vi "Robot_Arduino_1.vi"() -> ()   [LabVIEW 2013]
uses:
  <vilib>/Utility/inputDevices.llb/closeJoystick.vi
  <vilib>/LabVIEW Hacker/LINX/LVH-LINX.lvlib
panel:
  out "Ultrasonic":dbl
  out "Switch":bool
  in  "Serial Port":refnum<visa-resource-name>
  in  "stop":bool
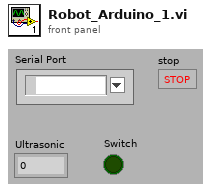
[diagram p1: front panel]
types:
  T1 = typedef "LVH-LINX.lvlib/LINX Ref.ctl" = cluster{"Platform":T2, "Interface":T3, "LINX Device Config":T4}
  T2 = typedef "LVH-LINX.lvlib/Platform.ctl" = enum16{"LINX", "myRIO"}
  T3 = typedef "LVH-LINX.lvlib/Interface.ctl" = enum16{"Serial", "TCP"}
  T4 = typedef "LVH-LINX.lvlib/Device.lvlib/LINX Device Config.ctl" = cluster{"Interface":T3, "COM Port":refnum<visa-resource-name>, "TCP Configuration":T5, "Device Family":T6, "Device ID":u8, "Device Name":string, "TCP Ref":refnum<k5>}
  T5 = typedef "LVH-LINX.lvlib/Device.lvlib/TCP Config.ctl" = cluster{"IP Address":string, "Port":u16}
  T6 = typedef "LVH-LINX.lvlib/Device Family.ctl" = enum8{"National Instruments", "Digilent", "Arduino"}
  T7 = cluster{"A":bool, "B":bool, "X":bool, " Y":bool, "Left_Trigger":dbl, "Right_Trigger ":dbl, "LB":bool, " RB":bool, "Left_Thumb_Button":bool, "Right_Thumb_Button":bool, "Stop_Back":bool, "Start":bool, "X_Axis_Left":dbl, "Y_Axis_Left":dbl, "X_Axis_Right":dbl, "Y_Axis_Right":dbl}
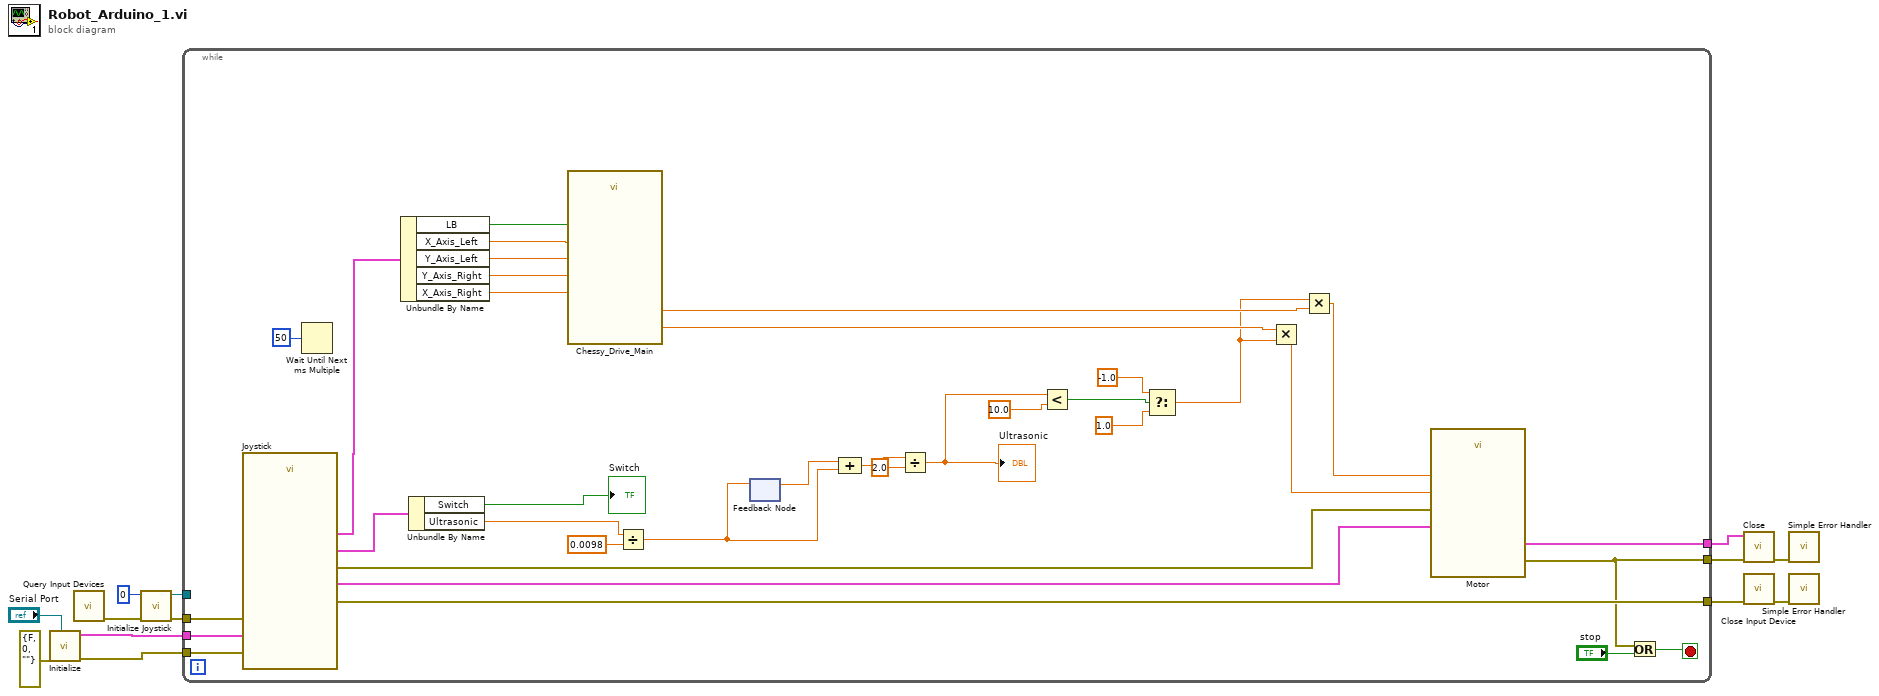
[diagram p0: block diagram]
diagram:
  n1 = call <vilib>:"Initialize.vi"("Serial Port"="Serial Port", "Error In"=errorcluster {"status"=FALSE, "code"=0, "source"=""}) -> ("Error Out"=w4:errorcluster, "LINX Ref"=w3:T1)  [unwired: 7 in, 1 out]
  n2 = call <vilib>:"Query Input Devices.vi"() -> ("error out"=w9:errorcluster)  [unwired: 1 in, 10 out]
  n3 = call <vilib>:"Initialize Joystick.vi"("error in (no error)"=w9, "device index"=0) -> ("error out"=w11:errorcluster, "device ID"=w12:refnum<k1>)  [unwired: 8 out]
  n4 = while {
    tunnel: w12 -> [_]
    tunnel: w11 -> [w48]
    tunnel: [w47] -> w10
    tunnel: w4 -> [w38]
    tunnel: w3 -> [w39]
    tunnel: [w42] -> w2
    tunnel: [w41] -> w1
    stop <- w44 stop-if-true
    n5 = call "Joystick.vi"("error in"=w48, "error in Linx"=w38, "LINX Ref"=w39) -> ("error out"=w47:errorcluster, "Signals"=w40:cluster{"Switch":bool, "Ultrasonic":dbl}, "Joystick"=w43:T7, "error out Linx"=w36:errorcluster, "LINX Ref"=w37:T1)  [unwired: 3 in, 1 out]
    n6 = Wait Until Next ms Multiple(millisecond multiple=u32 50) -> ()  [unwired: 1 out]
    n7 = Unbundle By Name(w43) -> ("LB"=w34:bool, "X_Axis_Left"=w33:dbl, "Y_Axis_Left"=w32:dbl, "Y_Axis_Right"=w31:dbl, "X_Axis_Right"=w30:dbl)
    n8 = Unbundle By Name(w40) -> ("Switch"=→"Switch":bool, "Ultrasonic"=w29:dbl)
    n9 = call "Chessy_Drive_Main.vi"("Speed_Main"=w32, "Turning_Main"=w30, "Speed_Limit"=w33, "Turning_Limit"=w31, "Quick_Turn"=w34) -> ("Left_Motor"=w17:dbl, "Right_Motor"=w18:dbl)  [unwired: 9 in]
    n10 = Divide(x=w29, y=0.0098) -> (x/y=w26:dbl)
    n11 = feedback-in #1(w26) -> ()
    n12 = feedback #1() -> (w27:dbl)  [unwired: 1 in]
    n13 = Compound Arithmetic op=ADD(w27, w26) -> (w25:dbl)
    n14 = Divide(x=w25, y=2.0) -> (x/y=w23:dbl)
    "Ultrasonic" <- w23
    n15 = Less?(x=w23, y=10.0) -> (x < y?=w21:bool)
    n16 = Select(t=-1.0, s=w21, f=1.0) -> (s? t:f=w16:dbl)
    n17 = Multiply(x=w18, y=w16) -> (x*y=w15:dbl)
    n18 = Multiply(x=w16, y=w17) -> (x*y=w14:dbl)
    n19 = call "Motor.vi"("error in Linx"=w36, "LINX Ref"=w37, "Motor_Right"=w15, "Motor_Left"=w14) -> ("error out"=w42:errorcluster, "LINX Resource"=w41:T1)  [unwired: 6 in]
    n20 = Or(x=w42, y="stop") -> (x .or. y?=w44:bool)
  }
  n21 = call <vilib>:"Close.vi"("Error In"=w2, "LINX Resource"=w1) -> ("Error Out"=w5:errorcluster)  [unwired: 8 in, 1 out]
  n22 = call-poly <vilib>:"Close Input Device.vi"("error in (no error)"=w10) -> ("error out"=w8:errorcluster)  [unwired: 1 in, 8 out]
  n23 = call <vilib>:"Simple Error Handler.vi"("error in (no error)"=w5) -> ()  [unwired: 4 in, 5 out]
  n24 = call <vilib>:"Simple Error Handler.vi"("error in (no error)"=w8) -> ()  [unwired: 1 in, 8 out]
